vi "i2c read.vi"(6 "bufferLength":i32, 7 "address":i32, 8 "error in (no error)":errorcluster, 9 "index":i32, 10 "result":cluster{"value":i32, "error":i32}, 11 "id":u32) -> (0 "error out":errorcluster, 1 "buffer":u8[](array[numeric]), 2 "result out":cluster{"value":i32, "error":i32}, 3 "id out":u32)   [LabVIEW 2014, in "BrainStem2_LabVIEW_Library.lvlib"]
doc: "aLIBEXPORT void __stdcall i2c_read ( unsigned int* id, struct Result* result, const int index , const int address, const int bufferLength, unsigned char * buffer ) ;"
uses:
  BrainStem2_LabVIEW_Library.lvlib
  BrainStem2_LabVIEW.dll
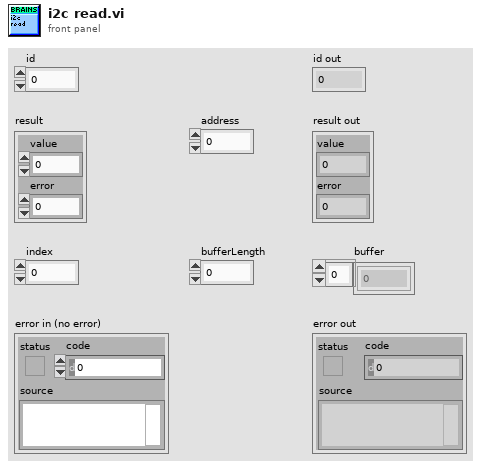
[diagram p1: front panel]
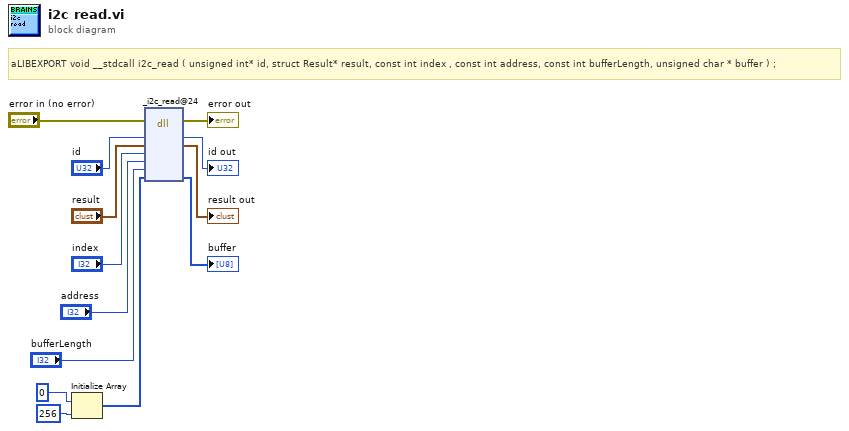
[diagram p0: block diagram]
diagram:
  # "aLIBEXPORT void __stdcall i2c_read ( unsigned int* id, struct Result* result, const int index , const int address, const int bufferLength, unsigned char * buffer ) ;"
  n1 = Initialize Array(u8 0 ("element"), 256 ("dimension size")) -> (w6:u8[])
  n2 = dll-call lib="C:/Users/mitch/Documents/development/acroname/software/acroname/aSource/BrainStem2/BrainStem2_LabVIEW/LabVIEW_2014_Distribution/BrainStem2_LabVIEW_w32/BrainStem2_LabVIEW.*" fn="_i2c_read@24"(error in="error in (no error)", "id"="id", "result"="result", "index"="index", "address"="address", "bufferLength"="bufferLength", "buffer"=w6) -> (error out=→"error out":errorcluster, "id"=→"id out":u32, "result"=→"result out":cluster{"value":i32, "error":i32}, "buffer"=→"buffer":u8[])  [unwired: 6 in, 1 out]
